vi "Advanced Specific Multiple Instruments.vi"() -> ()   [LabVIEW 2016]
doc: "Purpose: This example shows how to use specific channels ID and multiple connected instruments\nHardware setup: At least two Fluigent pressure modules"
uses:
  TypeDefs/fgt_INSTRUMENT_TYPE.ctl
  TypeDefs/fgt_CONTROLLER_INFO.ctl
  TypeDefs/fgt_CHANNEL_INFO.ctl
  fgt_SDK.lvlib
panel:
  out "Pressure 2":sgl format="%#_3g"
  out "Pressure 1":sgl format="%#_3g"
  out "error out":errorcluster
  out "Pressure channels info":T1[](array[typedef])
  out "Controllers channels info":T3[](array[typedef])
  out "Pressure channels count":u32
  out "Instruments count":i32
  out "Detected instruments":T4(array[cluster])
  # "Hit the \"Run\" button to read pressures"
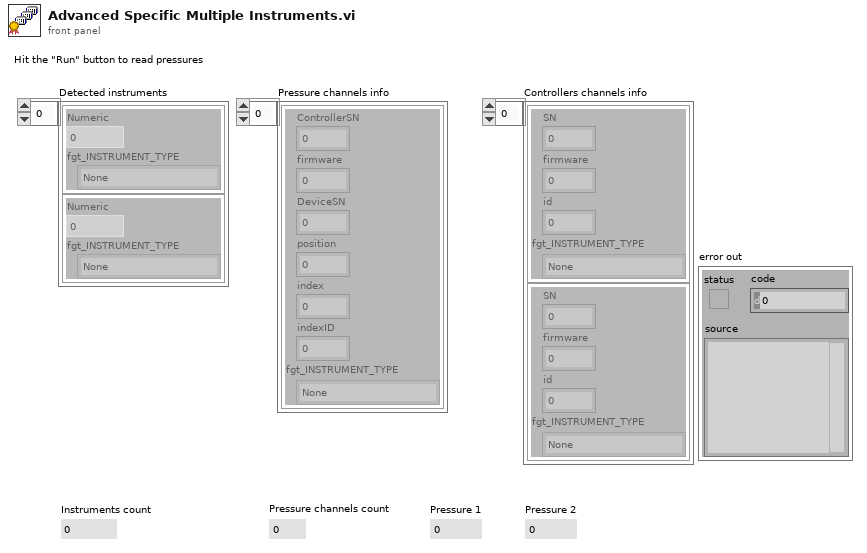
[diagram p1: front panel]
types:
  T1 = typedef "fgt_SDK.lvlib/fgt_CHANNEL_INFO.ctl" = cluster{"ControllerSN":u16, "firmware":u16, "DeviceSN":u16, "position":u32, "index":u32, "indexID":u32, "fgt_INSTRUMENT_TYPE":T2}
  T2 = typedef "fgt_SDK.lvlib/fgt_INSTRUMENT_TYPE.ctl" = enum32{"None", "MFCS", "MFCS_EZ", "FRP", "LineUP"}
  T3 = typedef "fgt_SDK.lvlib/fgt_CONTROLLER_INFO.ctl" = cluster{"SN":u16, "firmware":u16, "id":u32, "fgt_INSTRUMENT_TYPE":T2}
  T4 = cluster{"Numeric":u16, "fgt_INSTRUMENT_TYPE":T2}[]
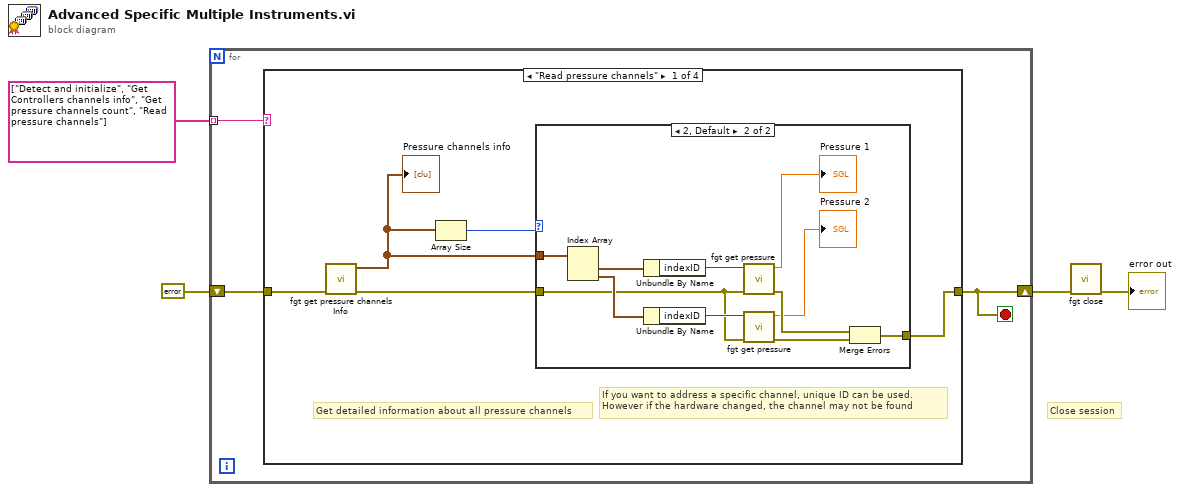
[diagram p0: block diagram]
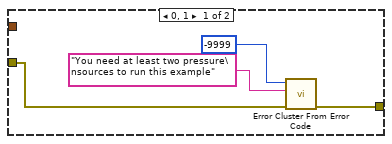
[diagram p2: hidden frame]
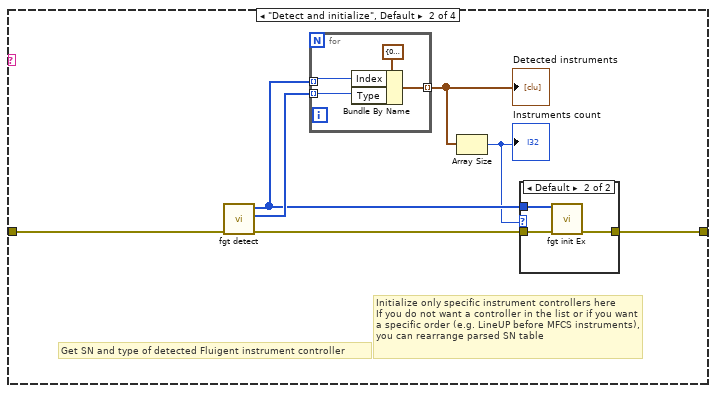
[diagram p3: hidden frame]
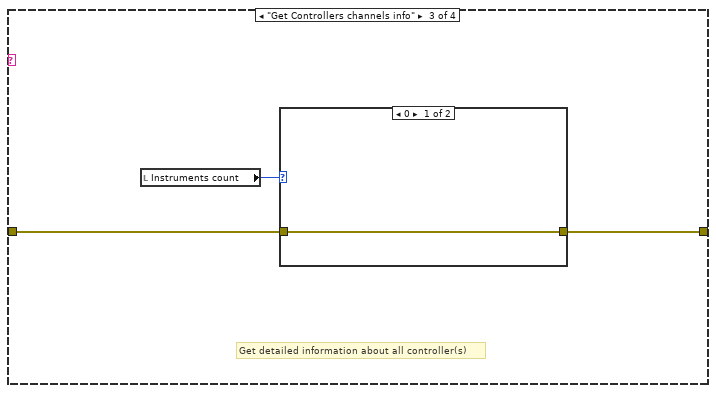
[diagram p5: hidden frame]
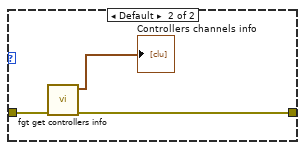
[diagram p6: hidden frame]
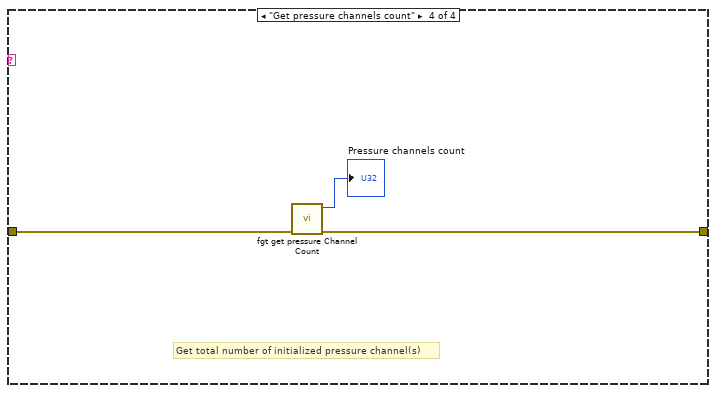
[diagram p7: hidden frame]
diagram:
  # "Close session"
  n1 = for {
    tunnel: string[] ["Detect and initialize", "Get Controllers channels info", "Get pressure channels count", "Read pressure channels"] -> [w7] mode=indexing
    shift-right: [w5] -> w1
    shift-left: errorcluster {"status"=FALSE, "code"=0, "source"=""} ("error in (no error)") -> [w6]
    stop <- w5 stop-if-true
    n2 = case shown="\"Read pressure channels\"" w7 {
      tunnel: w6 -> [w12 w30 w45 w51]
      tunnel: [w10 w29 w44 w50] -> w5
      frame "Read pressure channels" {
        # "If you want to address a specific channel, unique ID can be used. \nHowever if the hardware changed, the channel may not be found"
        # "Get detailed information about all pressure channels"
        n3 = call "fgt get pressure channels Info.vi"("error in (no error)"=w12) -> ("error out"=w11:errorcluster, "Pressure channels info"=w9:T1[])  [unwired: 9 in]
        "Pressure channels info" <- w9
        n4 = Array Size(array=w9) -> (size(s)=w8:i32)
        n5 = case shown="2, Default" w8 {
          tunnel: w11 -> [w13 w23]
          tunnel: [w14 w20] -> w10
          tunnel: w9 -> [_ w17]
          frame 0, 1 {
            n6 = call <vilib>:"Error Cluster From Error Code.vi"("error in (no error)"=w13, "error message (\"\")"="You need at least two pressure\nsources to run this example" ("error message (\"\")"), "error code (0)"=-9999) -> ("error out"=w14:errorcluster)  [unwired: 6 in]
          }
          frame 2, Default {
            n7 = Index Array(array=w17) -> (element #1=w24:T1, element #2=w27:T1)  [unwired: 2 in]
            n8 = Unbundle By Name(w24) -> ("indexID"=w25:u32)
            n9 = Unbundle By Name(w27) -> ("indexID"=w26:u32)
            n10 = call "fgt get pressure.vi"("error in (no error)"=w23, "pressureIndex"=w25) -> ("error out"=w22:errorcluster, "pressure out"=→"Pressure 1":sgl)  [unwired: 8 in]
            n11 = call "fgt get pressure.vi"("error in (no error)"=w23, "pressureIndex"=w26) -> ("error out"=w21:errorcluster, "pressure out"=→"Pressure 2":sgl)  [unwired: 8 in]
            n12 = Merge Errors(w22, w21) -> (w20:errorcluster)
          }
        }
      }
      frame "Detect and initialize", Default {
        # "Initialize only specific instrument controllers here\nIf you do not want a controller in the list or if you want a specific order (e.g. LineUP before MFCS instruments), you can\trearrange parsed SN table"
        # "Get SN and type of detected Fluigent instrument controller"
        n13 = call "fgt detect.vi"("error in (no error)"=w30) -> ("error out"=w32:errorcluster, "type out"=w33:T2[], "SN out"=w31:u16[])  [unwired: 8 in]
        n14 = for {
          tunnel: w31 -> [w42] mode=indexing
          tunnel: w33 -> [w41] mode=indexing
          tunnel: [w40] -> w34 mode=indexing
          n15 = Bundle By Name(cluster=cluster{"Index":u16, "Type":T2} {"Index"=0, "Type"=enum."None"}, "Index"=w42, "Type"=w41) -> (w40:cluster{"Index":u16, "Type":T2})
        }
        "Detected instruments" <- w34
        n16 = Array Size(array=w34) -> (size(s)=w28:i32)
        "Instruments count" <- w28
        n17 = case shown="Default" w28 {
          tunnel: w32 -> [w35 w38]
          tunnel: w31 -> [_ w37]
          tunnel: [w35 w36] -> w29
          frame 0 {
          }
          frame Default {
            n18 = call "fgt init Ex.vi"("error in (no error)"=w38, "SN"=w37) -> ("error out"=w36:errorcluster)  [unwired: 8 in, 1 out]
          }
        }
      }
      frame "Get Controllers channels info" {
        # "Get detailed information about all controller(s)"
        n19 = local read "Instruments count"() -> (w43:i32)
        n20 = case shown="0" w43 {
          tunnel: w45 -> [w46 w48]
          tunnel: [w46 w47] -> w44
          frame 0 {
          }
          frame Default {
            n21 = call "fgt get controllers info.vi"("error in (no error)"=w48) -> ("error out"=w47:errorcluster, "Controllers channels info"=→"Controllers channels info":T3[])  [unwired: 9 in]
          }
        }
      }
      frame "Get pressure channels count" {
        # "Get total number of initialized pressure channel(s)"
        n22 = call "fgt get pressure Channel Count.vi"("error in (no error)"=w51) -> ("error out"=w50:errorcluster, "nbPChan out"=→"Pressure channels count":u32)  [unwired: 9 in]
      }
    }
  }
  n23 = call "fgt close.vi"("error in (no error)"=w1) -> ("error out"=→"error out":errorcluster)  [unwired: 10 in]
